vi "FIFO Manager - Pre and Post.vi"(0 "Word In":u32, 7 "timeout in ms (-1)":i32, 11 "error in (no error)":errorcluster, 13 "Operation":T1) -> (8 "Timed Out":bool, 10 "Word Out":u32, 15 "error out":errorcluster)   [LabVIEW 2017, in "FPGA-SRL.lvlib"]
uses:
  FPGA-SRL.lvlib
  Type Defs/WSVCAP SHL FIFO Operation Enum.ctl
  <vilib>/rvi/DataTransferAndStorage/Container/XNode/niFpgaContainer.xnode
  <vilib>/rvi/FIFO/Fifo_Resource/nirvififoEmulationWrite.vi
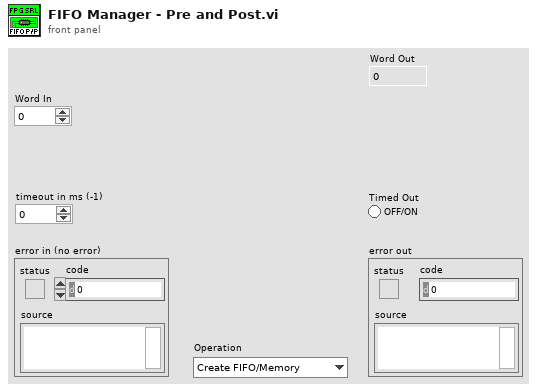
[diagram p1: front panel]
types:
  T1 = typedef "WSVCAP SHL FIFO Operation Enum.ctl" = enum16{"Create FIFO/Memory", "Get Write FIFO Status", "Get Read FIFO Status", "Put Element in Write", "Put Element in Read", "Get Element from Write", "Get Element from Read"}
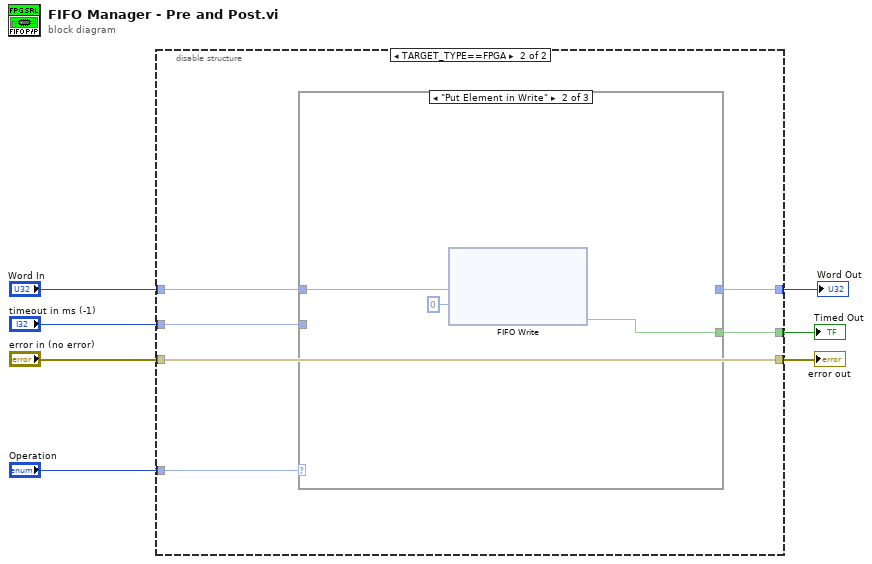
[diagram p0: block diagram]
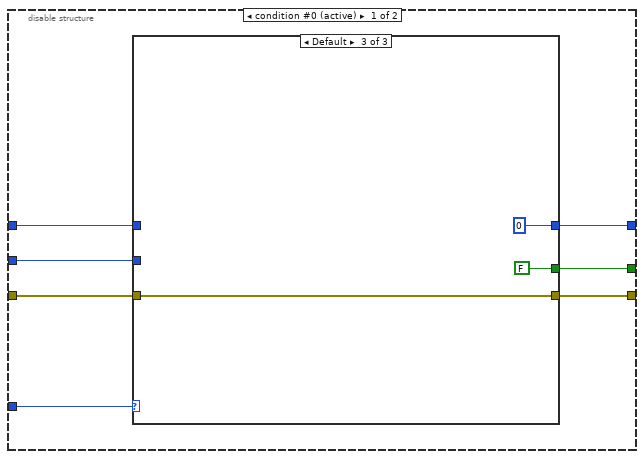
[diagram p2: hidden frame]
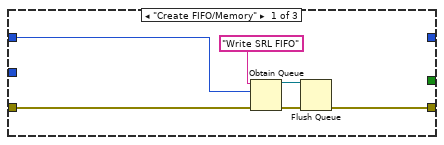
[diagram p3: hidden frame]
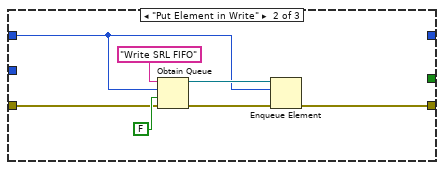
[diagram p4: hidden frame]
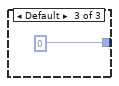
[diagram p6: hidden frame]
diagram:
  n1 = disable-structure shown="TARGET_TYPE==FPGA" {
    disable-tunnel: "Operation" -> [w14 w36]
    disable-tunnel: "error in (no error)" -> [w13 w31]
    disable-tunnel: [w12 w31] -> w5
    disable-tunnel: "Word In" -> [w11 w35]
    disable-tunnel: "timeout in ms (-1)" -> [w10 w34]
    disable-tunnel: [w9 w33] -> w2
    disable-tunnel: [w8 w32] -> w1
    frame condition #0 (active) {
      n2 = case shown="Default" w14 {
        tunnel: [w17 w22 w29] -> w12
        tunnel: w13 -> [w15 w23 w29]
        tunnel: w11 -> [w16 w21 _]
        tunnel: w10 -> [_ _ _]
        tunnel: [_ _ FALSE] -> w9
        tunnel: [_ _ u32 0 ("Word Out")] -> w8
        frame "Create FIFO/Memory" {
          n3 = Obtain Queue(name (unnamed)="Write SRL FIFO", element data type=w16, error in (no error)=w15) -> (queue out=w19:refnum<queue>, error out=w20:errorcluster)  [unwired: 2 in, 1 out]
          n4 = Flush Queue(queue=w19, error in (no error)=w20) -> (error out=w17:errorcluster)  [unwired: 2 out]
        }
        frame "Put Element in Write" {
          n5 = Obtain Queue(name (unnamed)="Write SRL FIFO", element data type=w21, create if not found? (T)=FALSE, error in (no error)=w23) -> (queue out=w26:refnum<queue>, error out=w27:errorcluster)  [unwired: 1 in, 1 out]
          n6 = Enqueue Element(queue=w26, element=w21, error in (no error)=w27) -> (error out=w22:errorcluster)  [unwired: 1 in, 2 out]
        }
        frame Default {
        }
      }
    }
    frame condition #1 {
      n7 = case shown="\"Put Element in Write\"" w36 {
        tunnel: w35 -> [_ w39 _]
        tunnel: w34 -> [_ _ _]
        tunnel: [_ w37 _] -> w33
        tunnel: [_ _ u32 0 ("Word Out")] -> w32
        frame "Create FIFO/Memory" {
        }
        frame "Put Element in Write" {
          n8 = xnode "FIFO Write"("Element"=w39, "Timeout"=0) -> ("Timed Out?"=w37:bool)  [unwired: 1 in, 1 out]
        }
        frame Default {
        }
      }
    }
  }
  "error out" <- w5
  "Timed Out" <- w2
  "Word Out" <- w1
